vi "Discover Node Connections Using Tag Info.vi"(9 "Show Tag Labels?":bool, 10 "tag info":T2(array[cluster]), 11 "channel and node pairs":T3[](array[typedef])) -> (3 "node connections":string[][](array[string]))   [LabVIEW 2015, in "GraphViz Mapping Visualizer.lvlib"]
uses:
  GraphViz Mapping Visualizer.lvlib
  Channel to Port Pair.ctl
  <vilib>/NI/Tag Bus/tag/Data Type.ctl
  <vilib>/NI/Tag Bus/tag/tag descriptor.lvclass
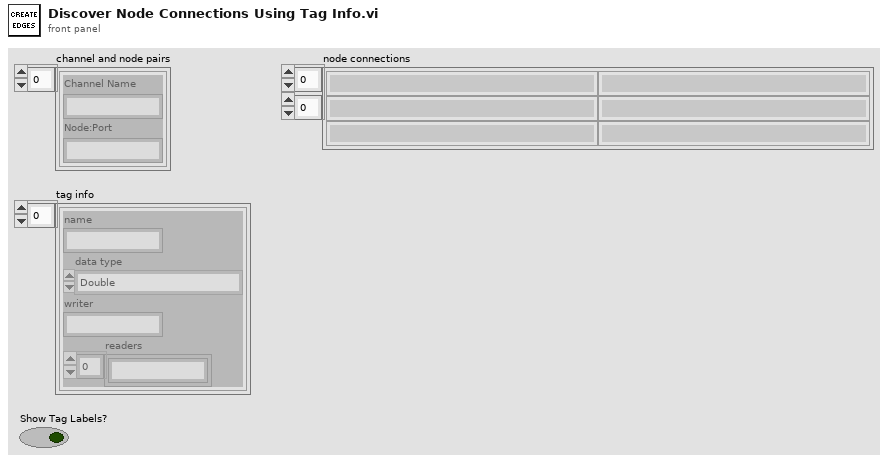
[diagram p1: front panel]
types:
  T1 = typedef "tag bus.lvlib/tag descriptor.lvclass/Data Type.ctl" = enum16{"Double", "Single", "I64", "I32", "I16", "I8", "U64", "U32", "U16", "U8", "Boolean", "String", "Array of Double", "Array of Single", "Array of I64", "Array of I32", "Array of I16", "Array of I8", "Array of U64", "Array of U32", "Array of U16", "Array of U8", "Array of Boolean", "Array of String"}
  T2 = cluster{"name":string, "data type":T1, "writer":string, "readers":string[]}[]
  T3 = typedef "GraphViz Mapping Visualizer.lvlib/Channel to Port Pair.ctl" = cluster{"Channel Name":string, "Node:Port":string}
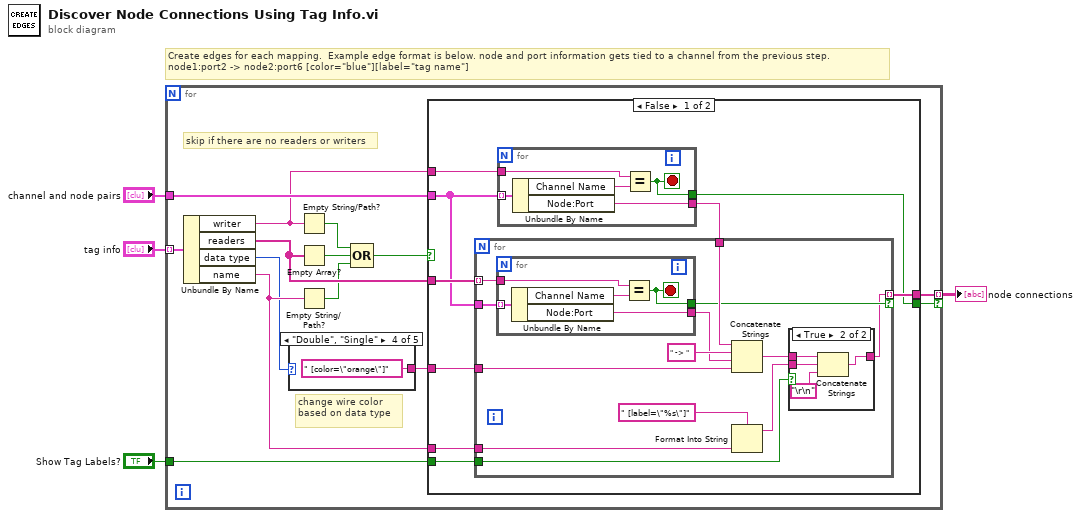
[diagram p0: block diagram]
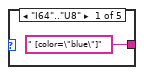
[diagram p2: hidden frame]
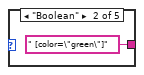
[diagram p3: hidden frame]
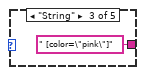
[diagram p4: hidden frame]
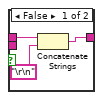
[diagram p6: hidden frame]
diagram:
  # "Create edges for each mapping.  Example edge format is below. node and port information gets tied to a channel from the previous step.\nnode1:port2 -> node2:port6 [color=\"blue\"][label=\"tag name\"]"
  n1 = for {
    tunnel: "channel and node pairs" -> [w16]
    tunnel: [w15] -> w3 mode=indexing if=w14
    tunnel: "Show Tag Labels?" -> [w13]
    tunnel: "tag info" -> [w12] mode=indexing
    # "change wire color based on data type"
    # "skip if there are no readers or writers"
    n2 = Unbundle By Name(w12) -> ("writer"=w11:string, "readers"=w10:string[], "data type"=w5:T1, "name"=w8:string)
    n3 = case shown="\"Double\", \"Single\"" w5 {
      tunnel: [" [color=\"blue\"]" ("string") " [color=\"green\"]" ("string") " [color=\"pink\"]" ("string") " [color=\"orange\"]" ("string") _] -> w6
      frame "I64".."U8" {
      }
      frame "Boolean" {
      }
      frame "String" {
      }
      frame "Double", "Single" {
      }
      frame Default {
      }
    }
    n4 = Empty String/Path?(string/path=w11) -> (empty?=w9:bool)
    n5 = Empty Array?(array=w10) -> (empty?=w18:bool)
    n6 = Empty String/Path?(string/path=w8) -> (empty?=w7:bool)
    n7 = Compound Arithmetic op=OR(w9, w18, w7) -> (w17:bool)
    n8 = case shown="False" w17 {
      tunnel: w16 -> [w30 _]
      tunnel: w10 -> [w31 _]
      tunnel: w11 -> [w29 _]
      tunnel: w8 -> [w27 _]
      tunnel: [w26 _] -> w15
      tunnel: [w25 _] -> w14
      tunnel: w13 -> [w24 _]
      tunnel: w6 -> [w23 _]
      frame False {
        n9 = for {
          tunnel: w29 -> [w34]
          tunnel: w30 -> [w36] mode=indexing
          tunnel: [w33] -> w25
          tunnel: [w32] -> w28
          stop <- w33 stop-if-true
          n10 = Unbundle By Name(w36) -> ("Channel Name"=w35:string, "Node:Port"=w32:string)
          n11 = Equal?(x=w34, y=w35) -> (x = y?=w33:bool)
        }
        n12 = for {
          tunnel: w31 -> [w49] mode=indexing
          tunnel: w30 -> [w48]
          tunnel: w28 -> [w47]
          tunnel: w27 -> [w44]
          tunnel: [w38] -> w26 mode=indexing if=w42
          tunnel: w24 -> [w41]
          tunnel: w23 -> [w37]
          n13 = for {
            tunnel: w49 -> [w59]
            tunnel: w48 -> [w61] mode=indexing
            tunnel: [w58] -> w42
            tunnel: [w57] -> w43
            stop <- w58 stop-if-true
            n14 = Unbundle By Name(w61) -> ("Channel Name"=w60:string, "Node:Port"=w57:string)
            n15 = Equal?(x=w59, y=w60) -> (x = y?=w58:bool)
          }
          n16 = Concatenate Strings(w47, " -> " ("string"), w43, w37) -> (w39:string)
          n17 = Format Into String(format string=" [label=\"%s\"]" ("string"), w44) -> (resulting string=w40:string)  [unwired: 2 in, 1 out]
          n18 = case shown="True" w41 {
            tunnel: w40 -> [_ w55]
            tunnel: w39 -> [w52 w56]
            tunnel: [w50 w54] -> w38
            frame False {
              n19 = Concatenate Strings(w52, "\r\n") -> (w50:string)
            }
            frame True {
              n20 = Concatenate Strings(w56, w55, "\r\n") -> (w54:string)
            }
          }
        }
      }
      frame True {
      }
    }
  }
  "node connections" <- w3
